vi "设定发布者.lvclass.vi"(8 "error in (no error)":errorcluster caption="错误输入（无错误）", 10 "数据采集.lvclass":refnum<class "数据采集.lvclass">, 11 "订阅者接口输入":refnum<class "订阅者接口.lvclass">) -> (0 "error out":errorcluster caption="错误输出", 3 "订阅者接口输出":refnum<class "订阅者接口.lvclass">)   [LabVIEW 2011, in "订阅者接口.lvclass"]
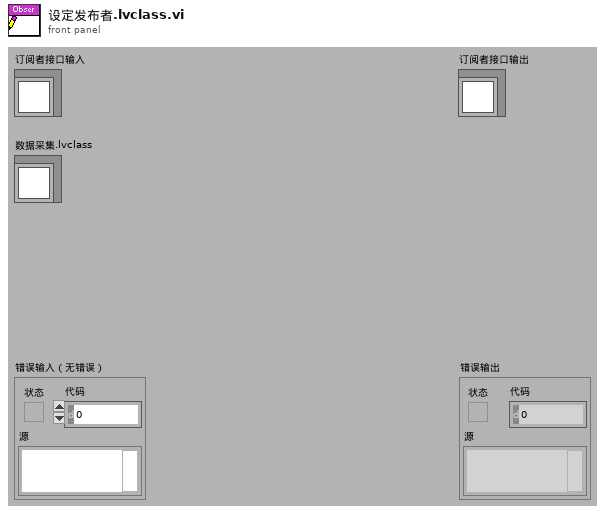
[diagram p1: front panel]
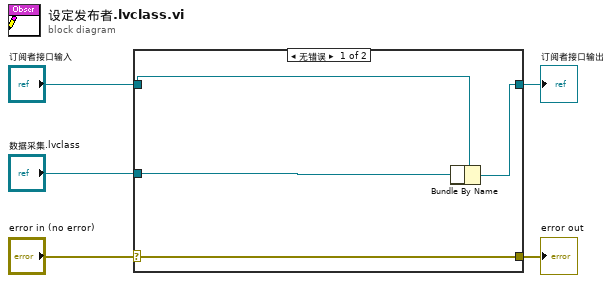
[diagram p0: block diagram]
diagram:
  n1 = case shown="无错误" "error in (no error)" {
    selector: "error in (no error)" -> [w9 w10]
    tunnel: [w9 w10] -> w4
    tunnel: [w7 w11] -> w2
    tunnel: "订阅者接口输入" -> [w8 w11]
    tunnel: "数据采集.lvclass" -> [w6 _]
    frame No Error {
      n2 = Bundle By Name(cluster=w8, w6) -> (w7:refnum<class "订阅者接口.lvclass">)
    }
    frame Error {
    }
  }
  "error out" <- w4
  "订阅者接口输出" <- w2
